vi "Constants.vi"() -> ()   [LabVIEW 2017, in "Untitled Project 1 Shared.lvlib"]
doc: "Use this Global VI to access the GUIDs assigned to the page resources of the Custom Device."
uses:
  Untitled Project 1 Shared.lvlib
panel:
  in  "Tab Control":enum32{"GUIDS", "Constants", "Properties"}(tab)
  in  "test":string="4f9117db-c222-415b-b593-b51a0972ce56"
  in  "Untitled Project 1":string="608488b5-938b-464d-bdde-e505747259ec"
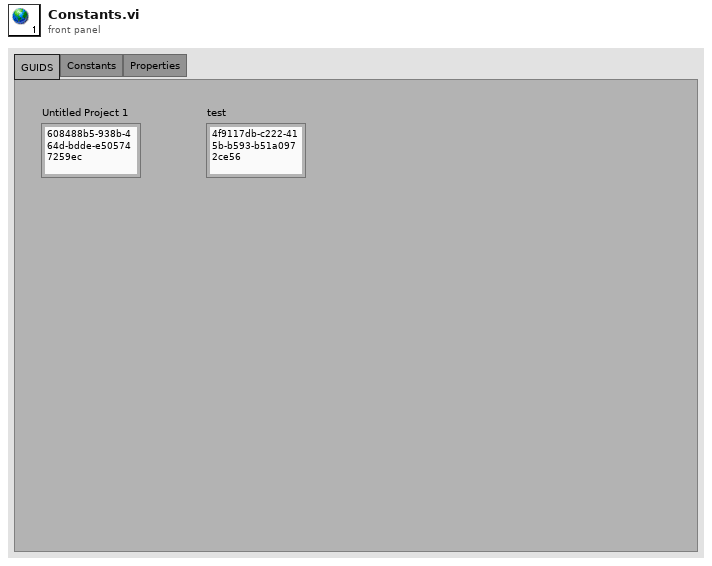
[diagram p1: front panel]
diagram:
